vi "Two Character Display (improved).vi"() -> ()   [LabVIEW 2014]
panel:
  out "Minute Ones":bool[](array[boolean])
  out "Minute Tens":bool[](array[boolean])
  out "Second Tens":bool[](array[boolean])
  out "Second Ones":bool[](array[boolean])
  in  "Stop Button":bool
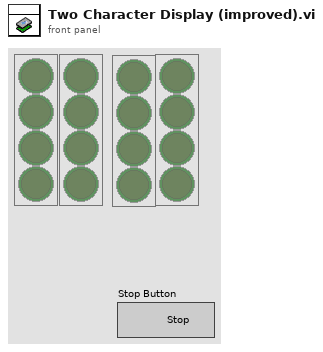
[diagram p1: front panel]
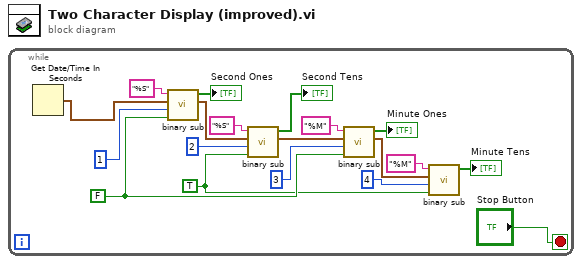
[diagram p0: block diagram]
diagram:
  n1 = while {
    stop <- "Stop Button" stop-if-true
    w8 = TRUE ("Tens?")
    w9 = FALSE ("Tens?")
    n2 = Get Date/Time In Seconds() -> (seconds since 1Jan1904=w1:timestamp)
    n3 = call "binary sub.vi"("Tens?"=w9, "order"=u8 1, "Time Stamp"=w1, "time format string (%c)"="%S") -> ("Time Stamp 2"=w15:timestamp, "Array"=→"Second Ones":bool[])  [unwired: 6 in]
    n4 = call "binary sub.vi"("Tens?"=w8, "order"=u8 2, "Time Stamp"=w15, "time format string (%c)"="%S") -> ("Time Stamp 2"=w14:timestamp, "Array"=→"Second Tens":bool[])  [unwired: 6 in]
    n5 = call "binary sub.vi"("Tens?"=w9, "order"=u8 3, "Time Stamp"=w14, "time format string (%c)"="%M") -> ("Time Stamp 2"=w13:timestamp, "Array"=→"Minute Ones":bool[])  [unwired: 6 in]
    n6 = call "binary sub.vi"("Tens?"=w8, "order"=u8 4, "Time Stamp"=w13, "time format string (%c)"="%M") -> ("Array"=→"Minute Tens":bool[])  [unwired: 6 in, 1 out]
  }
